vi "NISE.remote.Read Dev.HardwareVersion.vi"(8 "error in (no error)":errorcluster, 11 "SLSC Remote in":refnum<class "SLSC Interface.lvclass">) -> (0 "error out":errorcluster, 2 "Dev.HardwareVersion":string, 3 "SLSC Remote out":refnum<class "SLSC Interface.lvclass">)   [LabVIEW 2016, in "SLSC Interface.lvclass"]
uses:
  SLSC Interface Class/SLSC Interface.lvclass
  <vilib>/NI/JSON Support for LabVIEW/JSON Value/JSON Value.lvclass
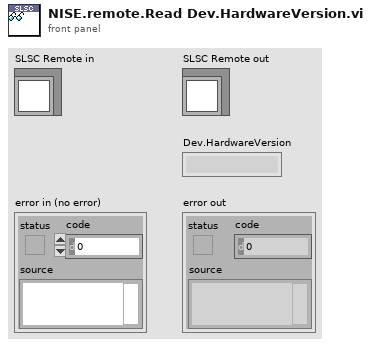
[diagram p1: front panel]
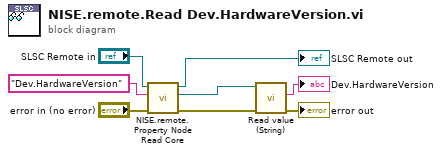
[diagram p0: block diagram]
diagram:
  n1 = call "NISE.remote.Property Node Read Core.vi"("error in (no error)"="error in (no error)", "property"="Dev.HardwareVersion", "SLSC Remote in"="SLSC Remote in") -> ("error out"=w4:errorcluster, "JSON Value out"=w1:refnum<class "JSON Value.lvclass">, "SLSC Remote out"=→"SLSC Remote out":refnum<class "SLSC Interface.lvclass">)  [unwired: 6 in]
  n2 = call <vilib>:"Read value (String).vi"("error in (no error)"=w4, "JSON String in"=w1) -> ("error out"=→"error out":errorcluster, "value"=→"Dev.HardwareVersion":string)  [unwired: 8 in]
